vi "pointBetweenTwoOthers.vi"(7 "Query":dbl[](array[numeric]), 8 "error in (no error)":errorcluster, 9 "P2":dbl[](array[numeric]), 10 "P1":dbl[](array[numeric]), 11 "Utilities in":refnum<class "Utilities.lvclass">) -> (0 "error out":errorcluster, 2 "queryBetweenP1P2":bool, 3 "Utilities out":refnum<class "Utilities.lvclass">)   [LabVIEW 2021, in "Utilities.lvclass"]
uses:
  Utilities.lvclass
  <vilib>/Analysis/coordinate.llb/2D Cartesian Coordinate Rotation (Scalar).vi
  <vilib>/Analysis/NI_AALPro.lvlib
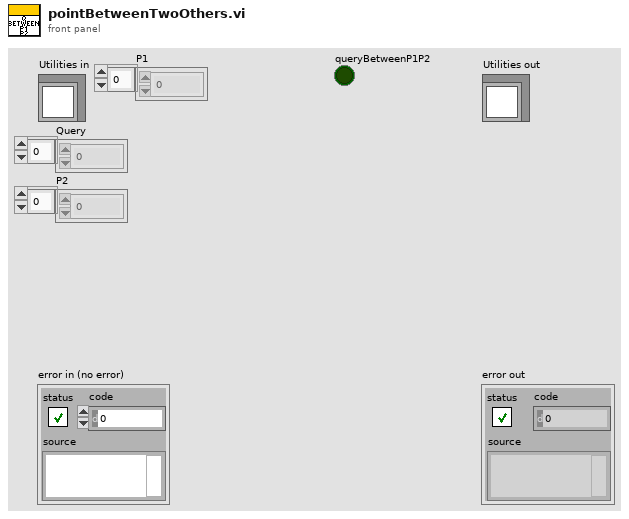
[diagram p1: front panel]
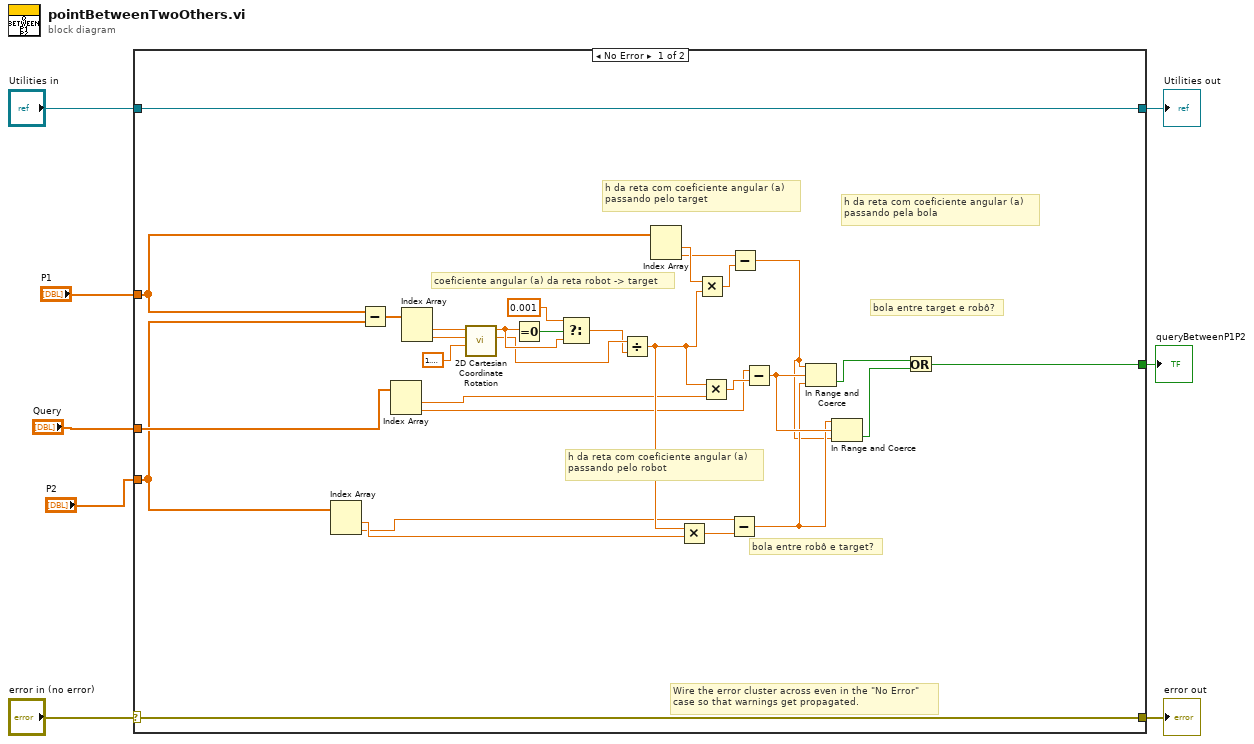
[diagram p0: block diagram]
diagram:
  n1 = case shown="No Error" "error in (no error)" {
    selector: "error in (no error)" -> [w37 w40]
    tunnel: [w37 w40] -> w7
    tunnel: [w38 w39] -> w5
    tunnel: "Utilities in" -> [w38 w39]
    tunnel: "Query" -> [w16 _]
    tunnel: "P1" -> [w13 _]
    tunnel: "P2" -> [w12 _]
    tunnel: [w9 _] -> w1
    frame No Error {
      # "bola entre target e robô?"
      # "bola entre robô e target?"
      # "h da reta com coeficiente angular (a)\npassando pelo robot"
      # "h da reta com coeficiente angular (a)\npassando pela bola"
      # "h da reta com coeficiente angular (a)\npassando pelo target"
      # "coeficiente angular (a) da reta robot -> target"
      # "Wire the error cluster across even in the \"No Error\"\ncase so that warnings get propagated."
      n2 = Index Array(array=w12) -> (element #1=w11:dbl, element #2=w10:dbl)  [unwired: 2 in]
      n3 = Subtract(x=w13, y=w12) -> (x-y=w36:dbl[])
      n4 = Index Array(array=w16) -> (element #1=w15:dbl, element #2=w14:dbl)  [unwired: 2 in]
      n5 = Index Array(array=w36) -> (element #1=w35:dbl, element #2=w34:dbl)  [unwired: 2 in]
      n6 = call-poly <vilib>:"2D Cartesian Coordinate Rotation.vi"("theta"=1.5707963267948966, "y"=w34, "x"=w35) -> ("y out"=w29:dbl, "x out"=w30:dbl)  [unwired: 6 in, 1 out]
      n7 = Equal To 0?(x=w30) -> (x = 0?=w32:bool)
      n8 = Select(t=0.001, s=w32, f=w30) -> (s? t:f=w28:dbl)
      n9 = Divide(x=w29, y=w28) -> (x/y=w23:dbl)
      n10 = Index Array(array=w13) -> (element #1=w27:dbl, element #2=w26:dbl)  [unwired: 2 in]
      n11 = Multiply(x=w23, y=w11) -> (x*y=w22:dbl)
      n12 = Multiply(x=w27, y=w23) -> (x*y=w25:dbl)
      n13 = Multiply(x=w23, y=w15) -> (x*y=w24:dbl)
      n14 = Subtract(x=w10, y=w22) -> (x-y=w19:dbl)
      n15 = Subtract(x=w26, y=w25) -> (x-y=w18:dbl)
      n16 = Subtract(x=w14, y=w24) -> (x-y=w20:dbl)
      n17 = In Range and Coerce(upper limit=w18, x=w20, lower limit=w19) -> (In Range?=w21:bool)  [unwired: 1 out]
      n18 = In Range and Coerce(upper limit=w19, x=w20, lower limit=w18) -> (In Range?=w17:bool)  [unwired: 1 out]
      n19 = Or(x=w21, y=w17) -> (x .or. y?=w9:bool)
    }
    frame Error {
    }
  }
  "error out" <- w7
  "Utilities out" <- w5
  "queryBetweenP1P2" <- w1
